vi "Incremental PCA.vi"() -> ()   [LabVIEW 2020]
doc: "Incremental principal component analysis (IPCA) is typically used as a replacement for principal component analysis (PCA) when the dataset to be decomposed is too large to fit in memory. IPCA builds a low-rank approximation for the input data using an amount of memory which is independent of the number of input data samples. It is still dependent on the input data features, but changing the batch size allows for control of memory usage.\n\nThis example serves as a visual check that IPCA is able to find a similar projection of the data to PCA (to a sign flip), while only processing a few samples at a time. This can be considered a “toy example”, as IPCA is intended for large datasets which do not fit in main memory, requiring incremental approaches."
uses:
  Model/Unsupervised/Decomposition/IncrementalPCA/Controls/incremental_pca_params.ctl
  Model/Unsupervised/Decomposition/PCA/Controls/pca_params.ctl
  Display/Classification/2D/Predicted/Controls/PredictedParameter.ctl
  Display/_Controls/Style.ctl
  Model/Unsupervised/Decomposition/IncrementalPCA/IncrementalPCA.lvclass
  C:/Users/cipop/TDF Dropbox/2_Technologies de France/1 - Services et Etudes/PLAIY/2 - DEV/PLAIYLAB/code/Model/Model.lvclass
  Model/Unsupervised/Decomposition/PCA/PCA.lvclass
  Model/Unsupervised/Decomposition/IncrementalPCA/IncrementalPCA.vi
  Model/Unsupervised/Decomposition/PCA/PCA.vi
panel:
  out "Plot 2":cluster{"X":dbl[], "Y":dbl[]}[](graph) caption="PCA of iris dataset"
  out "error out":errorcluster
  in  "error in":errorcluster
  out "Plot":cluster{"X":dbl[], "Y":dbl[]}[](graph) caption="Incremental PCA  of iris dataset"
  in  "Local":T1
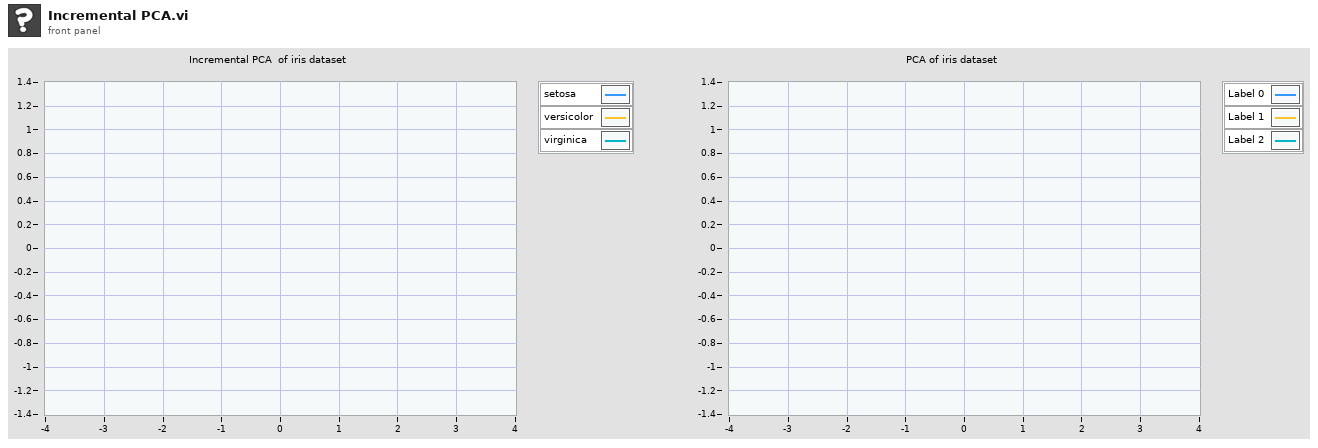
[diagram p1: front panel]
types:
  T1 = cluster{"X":dbl[][], "y":dbl[], "X_ipca":dbl[][], "X_pca":dbl[][]}
  T2 = typedef "incremental_pca_params.ctl" = cluster{"n_components":cluster{"n_components_type":string, "n_components_int":dbl}, "whiten":bool, "copy":bool, "batch_size":cluster{"batch_size_type":string, "batch_size_int":dbl}}
  T3 = typedef "pca_params.ctl" = cluster{"n_components":cluster{"n_components_type":string, "n_components_int":i32, "n_components_float":dbl}, "copy":bool, "whiten":bool, "svd_solver":string, "tol":dbl, "iterated_power":cluster{"iterated_power_type":string, "iterated_power_int":dbl}, "random_state":dbl}
  T4 = typedef "Style.ctl" = enum16{"Empty circle", "Full circle", "Empty square", "Full square", "Cross"}
  T5 = typedef "PredictedParameter.ctl" = cluster{"Plot":refnum<vi>, "Data":cluster{"X":dbl[][], "Predict":dbl[][]}, "Indexe":cluster{"X":i32, "Y":i32}, "Point Property":cluster{"Style":T4, "Label Color":u32[]}}
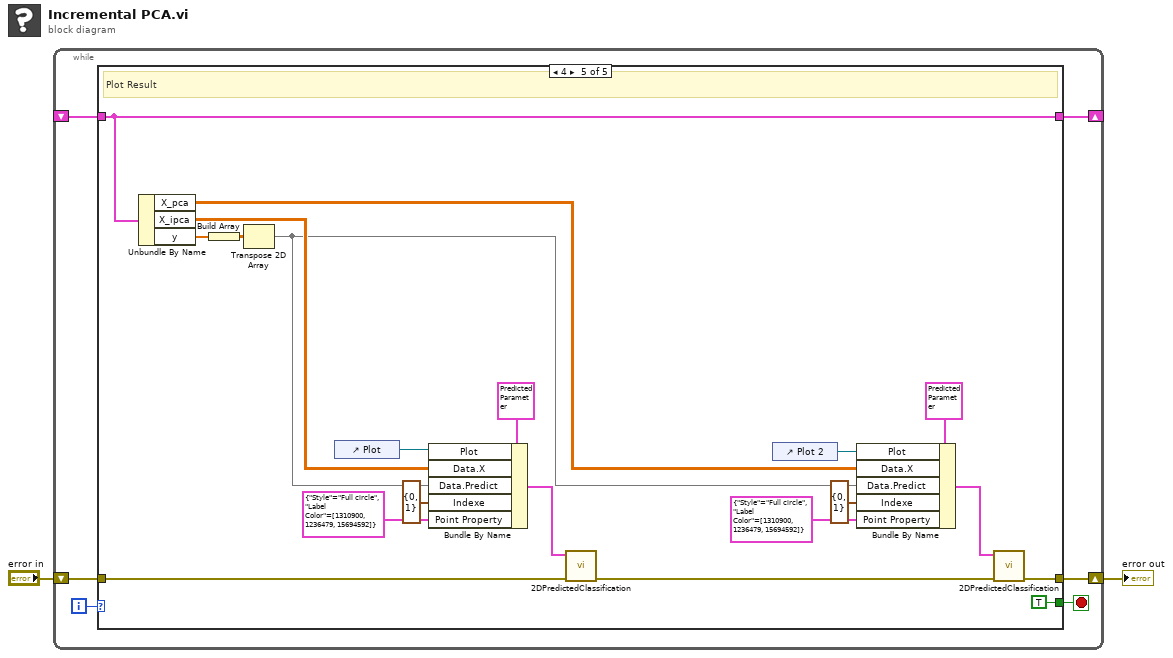
[diagram p0: block diagram]
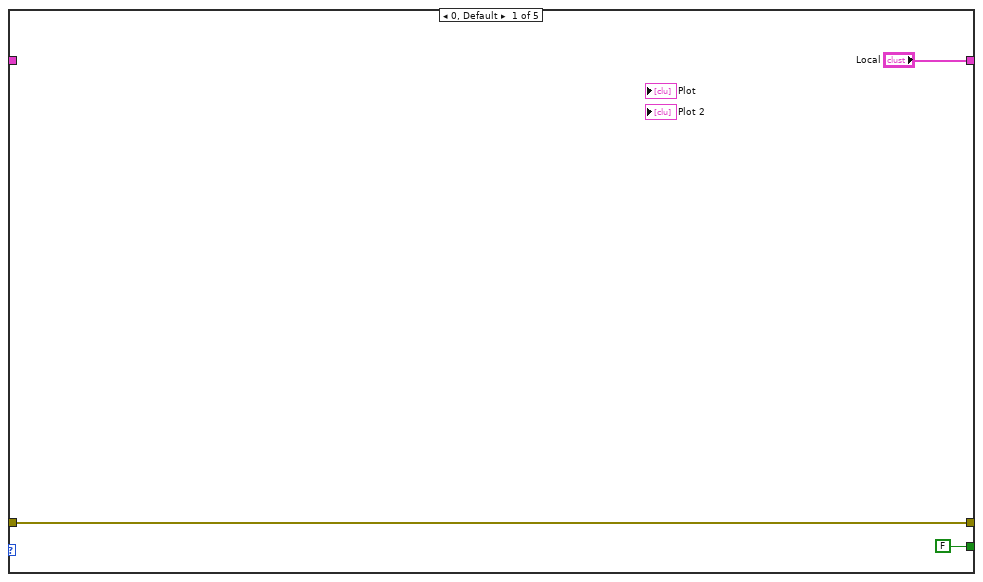
[diagram p2: hidden frame]
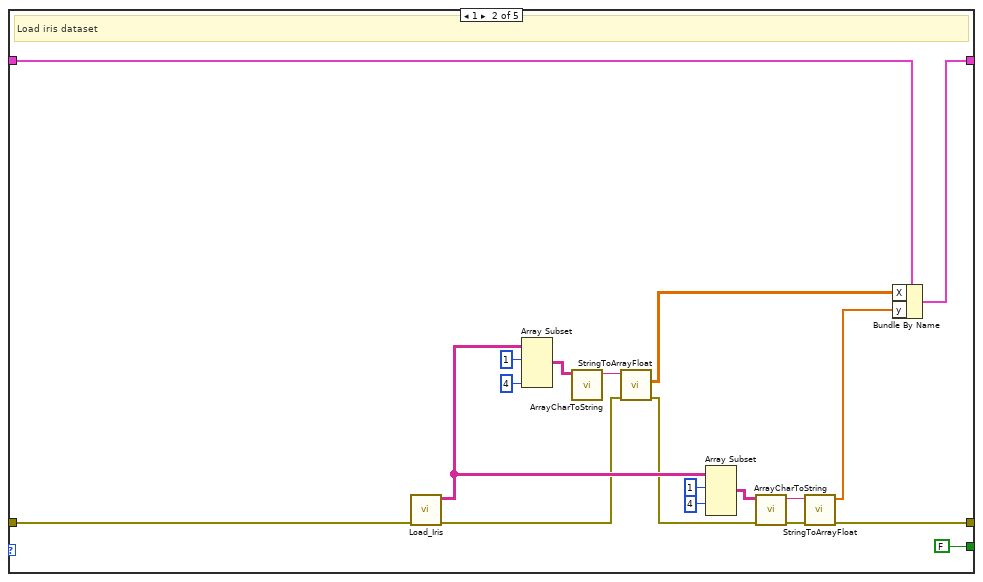
[diagram p3: hidden frame]
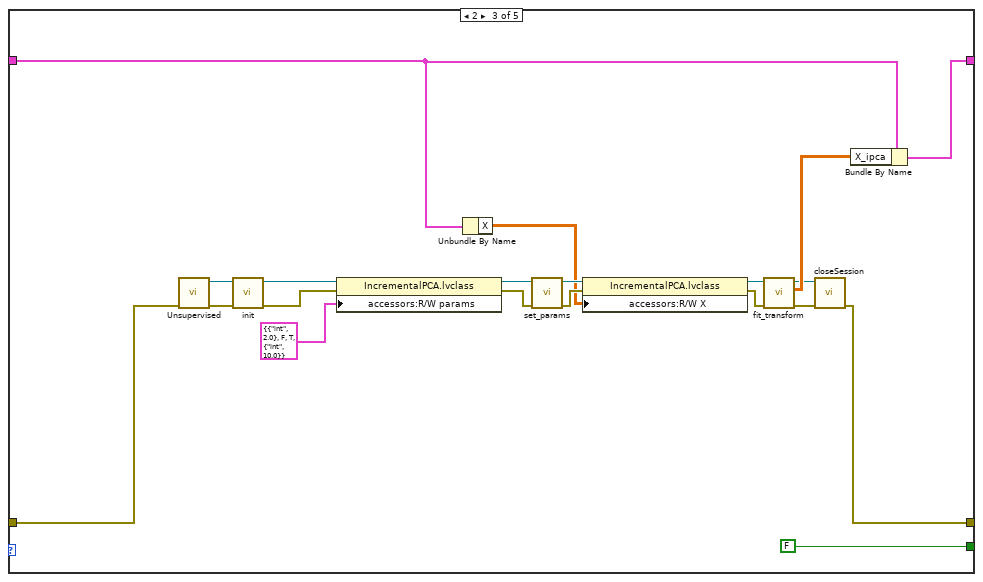
[diagram p4: hidden frame]
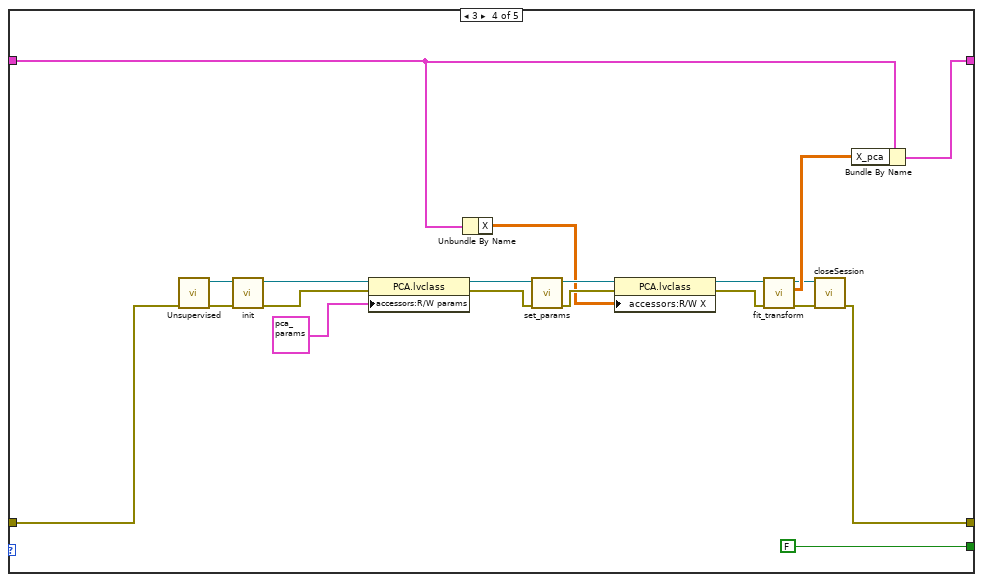
[diagram p5: hidden frame]
diagram:
  n1 = while {
    shift-right: [w6] -> w1
    shift-left: "error in" -> [w7]
    shift-right: [w5] -> _
    shift-left: _ -> [w4]
    i -> [w8]
    stop <- w3 stop-if-true
    n2 = case shown="4" w8 {
      tunnel: w7 -> [w10 w16 w38 w58 w86]
      tunnel: [w10 w13 w30 w51 w74] -> w6
      tunnel: ["Local" w27 w42 w62 w70] -> w5
      tunnel: w4 -> [_ w28 w43 w63 w70]
      tunnel: [FALSE FALSE FALSE FALSE TRUE] -> w3
      frame 0, Default {
      }
      frame 1 {
        # "Load iris dataset"
        n3 = call "Load_Iris.vi"("error in"=w16) -> ("error out"=w17:errorcluster, "Tableau"=w22:string[][])  [unwired: 9 in]
        n4 = Array Subset(array=w22, index (row)=1 ("index"), length (col)=4 ("length")) -> (w20:string[][])  [unwired: 2 in]
        n5 = call "ArrayCharToString.vi"("TAB"=w20) -> ("Instruction"=w21:string)  [unwired: 10 in]
        n6 = call "StringToArrayFloat.vi"("entrée d'erreur (pas d'erreur)"=w17, "Return value"=w21) -> ("error IO"=w14:errorcluster, "2DArray"=w15:dbl[][])  [unwired: 7 in, 1 out]
        n7 = Array Subset(array=w22, index (row)=1 ("index"), index (col)=4 ("index")) -> (w18:string[][])  [unwired: 2 in]
        n8 = call "ArrayCharToString.vi"("TAB"=w18) -> ("Instruction"=w19:string)  [unwired: 10 in]
        n9 = call "StringToArrayFloat.vi"("entrée d'erreur (pas d'erreur)"=w14, "Return value"=w19) -> ("error IO"=w13:errorcluster, "1DArray"=w12:dbl[])  [unwired: 7 in, 1 out]
        n10 = Bundle By Name(cluster=w28, "X"=w15, "y"=w12) -> (w27:T1)
      }
      frame 2 {
        n11 = call-poly "Unsupervised.vi"("error in"=w38) -> ("error out"=w39:errorcluster, "out"=w40:refnum<class "IncrementalPCA.lvclass">)  [unwired: 9 in]
        n12 = call-dynamic "init.vi"("error in (no error)"=w39, "Model en entrée"=w40) -> ("error out"=w44:errorcluster, "Model en sortie"=w48:refnum<class "IncrementalPCA.lvclass">)  [unwired: 8 in]
        n13 = property class="IncrementalPCA.lvclass"(reference=w48, error in=w44, "accessors:R/W params"=T2 {"n_components"={"n_components_type"="int", "n_components_int"=2.0}, "whiten"=FALSE, "copy"=TRUE, "batch_size"={"batch_size_type"="int", "batch_size_int"=10.0}} ("R/W params")) -> (reference out=w47:refnum<class "IncrementalPCA.lvclass">, error out=w41:errorcluster)
        n14 = Unbundle By Name(w43) -> ("X"=w34:dbl[][])
        n15 = call-dynamic "set_params.vi"("error in (no error)"=w41, "IncrementalPCA.lvclass 2"=w47) -> ("error out"=w45:errorcluster, "IncrementalPCA.lvclass"=w46:refnum<class "IncrementalPCA.lvclass">)  [unwired: 8 in]
        n16 = property class="IncrementalPCA.lvclass"(reference=w46, error in=w45, "accessors:R/W X"=w34) -> (reference out=w36:refnum<class "IncrementalPCA.lvclass">, error out=w35:errorcluster)
        n17 = call-dynamic "fit_transform.vi"("error in (no error)"=w35, "Decomposition.lvclass 2"=w36) -> ("error out"=w31:errorcluster, "X_new"=w33:dbl[][], "Decomposition.lvclass"=w32:refnum<class "IncrementalPCA.lvclass">)  [unwired: 7 in]
        n18 = call-dynamic "closeSession.vi"("error in"=w31, "Python en entrée"=w32) -> ("error out"=w30:errorcluster)  [unwired: 8 in, 1 out]
        n19 = Bundle By Name(cluster=w43, "X_ipca"=w33) -> (w42:T1)
      }
      frame 3 {
        n20 = call-poly "Unsupervised.vi"("error in"=w58) -> ("error out"=w59:errorcluster, "out"=w60:refnum<class "PCA.lvclass">)  [unwired: 9 in]
        n21 = call-dynamic "init.vi"("error in (no error)"=w59, "Model en entrée"=w60) -> ("error out"=w64:errorcluster, "Model en sortie"=w68:refnum<class "PCA.lvclass">)  [unwired: 8 in]
        n22 = property class="PCA.lvclass"(reference=w68, error in=w64, "accessors:R/W params"=T3 {"n_components"={"n_components_type"="int", "n_components_int"=2, "n_components_float"=0.0}, "copy"=TRUE, "whiten"=FALSE, "svd_solver"="auto", "tol"=0.0, "iterated_power"={"iterated_power_type"="auto", "iterated_power_int"=0.0}, "random_state"=0.0} ("R/W params")) -> (reference out=w67:refnum<class "PCA.lvclass">, error out=w61:errorcluster)
        n23 = Unbundle By Name(w63) -> ("X"=w55:dbl[][])
        n24 = call-dynamic "set_params.vi"("error in (no error)"=w61, "PCA.lvclass 2"=w67) -> ("error out"=w65:errorcluster, "PCA.lvclass"=w66:refnum<class "PCA.lvclass">)  [unwired: 8 in]
        n25 = property class="PCA.lvclass"(reference=w66, error in=w65, "accessors:R/W X"=w55) -> (reference out=w57:refnum<class "PCA.lvclass">, error out=w56:errorcluster)
        n26 = call-dynamic "fit_transform.vi"("error in (no error)"=w56, "Decomposition.lvclass 2"=w57) -> ("error out"=w52:errorcluster, "X_new"=w54:dbl[][], "Decomposition.lvclass"=w53:refnum<class "PCA.lvclass">)  [unwired: 7 in]
        n27 = call-dynamic "closeSession.vi"("error in"=w52, "Python en entrée"=w53) -> ("error out"=w51:errorcluster)  [unwired: 8 in, 1 out]
        n28 = Bundle By Name(cluster=w63, "X_pca"=w54) -> (w62:T1)
      }
      frame 4 {
        # "Plot Result"
        n29 = Unbundle By Name(w70) -> ("X_pca"=w72:dbl[][], "X_ipca"=w82:dbl[][], "y"=w84:dbl[])
        n30 = Build Array(w84) -> (w83:dbl[][])
        n31 = Transpose 2D Array(2D array=w83) -> (transposed array=w73:dbl[][])
        n32 = control-ref of="Plot"() -> (w85:refnum<vi>)
        n33 = Bundle By Name(cluster=T5 {"Plot"=refnum, "Data"={"X"=[], "Predict"=[]}, "Indexe"={"X"=0, "Y"=1}, "Point Property"={"Style"=enum."Full circle", "Label Color"=[8978528, 4367871, 1985280]}} ("Parameters"), "Plot"=w85, "Data.X"=w82, "Data.Predict"=w73, "Indexe"=cluster{"X":i32, "Y":i32} {"X"=0, "Y"=1}, "Point Property"=cluster{"Style":T4, "Label Color":u32[]} {"Style"=enum."Full circle", "Label Color"=[1310900, 1236479, 15694592]}) -> (w89:T5)
        n34 = call "2DPredictedClassification.vi"("error in"=w86, "Parameters"=w89) -> ("error out"=w75:errorcluster)  [unwired: 9 in]
        n35 = control-ref of="Plot 2"() -> (w71:refnum<vi>)
        n36 = Bundle By Name(cluster=T5 {"Plot"=refnum, "Data"={"X"=[], "Predict"=[]}, "Indexe"={"X"=0, "Y"=1}, "Point Property"={"Style"=enum."Full circle", "Label Color"=[8978528, 4367871, 1985280]}} ("Parameters"), "Plot"=w71, "Data.X"=w72, "Data.Predict"=w73, "Indexe"=cluster{"X":i32, "Y":i32} {"X"=0, "Y"=1}, "Point Property"=cluster{"Style":T4, "Label Color":u32[]} {"Style"=enum."Full circle", "Label Color"=[1310900, 1236479, 15694592]}) -> (w76:T5)
        n37 = call "2DPredictedClassification.vi"("error in"=w75, "Parameters"=w76) -> ("error out"=w74:errorcluster)  [unwired: 9 in]
      }
    }
  }
  "error out" <- w1
